vi "AutoDataDB.vi"() -> (3 "output cluster":T1)   [LabVIEW 2014]
uses:
  Common Code/AutonomousDBPacket.ctl
  commandCluster.ctl
  Robot Global Data.vi
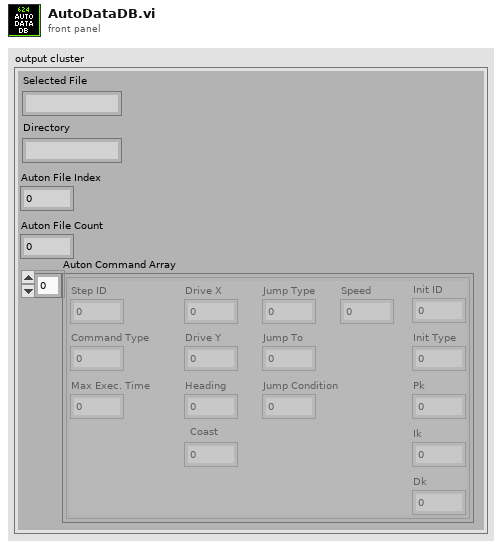
[diagram p1: front panel]
types:
  T1 = typedef "AutonomousDBPacket.ctl" = cluster{"Selected File":string, "Directory":string, "Auton File Index":i32, "Auton File Count":i32, "Auton Command Array":T2[]}
  T2 = typedef "commandCluster.ctl" = cluster{"Step ID":i32, "Command Type":i32, "Drive X":dbl, "Drive Y":dbl, "Heading":dbl, "Max Exec. Time":u32, "Jump Type":i32, "Jump To":i32, "Jump Condition":i32, "Coast":i32, "Speed":dbl, "Init ID":i32, "Init Type":i32, "Pk":dbl, "Ik":dbl, "Dk":dbl}
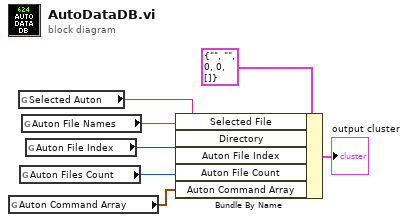
[diagram p0: block diagram]
diagram:
  n1 = global read "Robot Global Data.vi" "Auton Command Array"() -> (w1:T2[])
  n2 = global read "Robot Global Data.vi" "Selected Auton"() -> (w5:string)
  n3 = global read "Robot Global Data.vi" "Auton Files Count"() -> (w7:i32)
  n4 = global read "Robot Global Data.vi" "Auton File Names"() -> (w4:string)
  n5 = global read "Robot Global Data.vi" "Auton File Index"() -> (w6:i32)
  n6 = Bundle By Name(cluster=T1 {"Selected File"="", "Directory"="", "Auton File Index"=0, "Auton File Count"=0, "Auton Command Array"=[]} ("Autonomous"), "Selected File"=w5, "Directory"=w4, "Auton File Index"=w6, "Auton File Count"=w7, "Auton Command Array"=w1) -> (→"output cluster":T1)
